vi "append to kpro data array 2016.vi"(6 "Cluster in":T1, 7 "Zeroed Pressure":dbl format="%.2f", 9 "Flow":dbl, 10 "Corrected Array in":dbl[][](array[numeric]), 11 "Feet of\nStainless to be\nUsed (Count) in":i32) -> (1 "IK":dbl, 2 "Array":dbl[][](array[numeric]), 3 "Cluster out 2":T1)   [LabVIEW 2016]
uses:
  Waterloo DAQ/controls/Kpro hydraulic measurement cluster.ctl
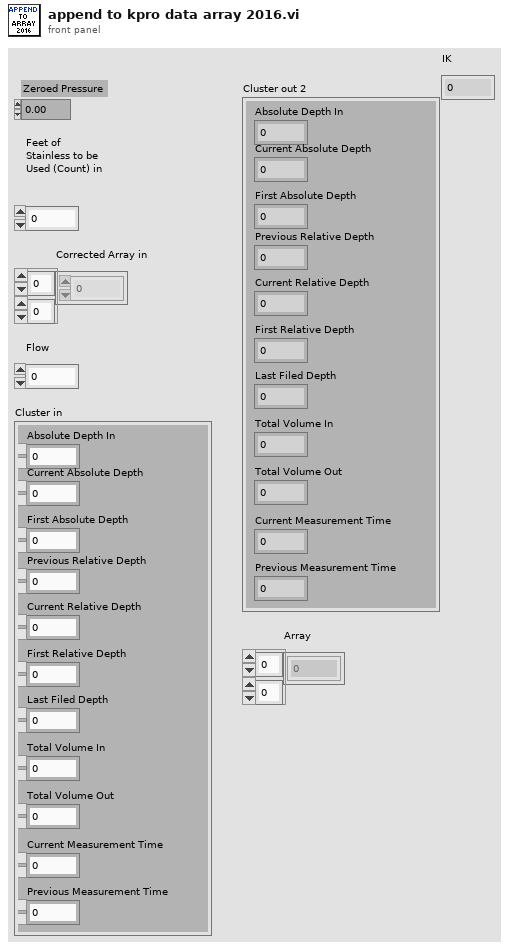
[diagram p1: front panel]
types:
  T1 = typedef "Kpro hydraulic measurement cluster.ctl" = cluster{"Absolute Depth In":dbl, "Current Absolute Depth":dbl, "First Absolute Depth":dbl, "Previous Relative Depth":dbl, "Current Relative Depth":dbl, "First Relative Depth":dbl, "Last Filed Depth":dbl, "Total Volume In":dbl, "Total Volume Out":dbl, "Current Measurement Time":dbl, "Previous Measurement Time":dbl}
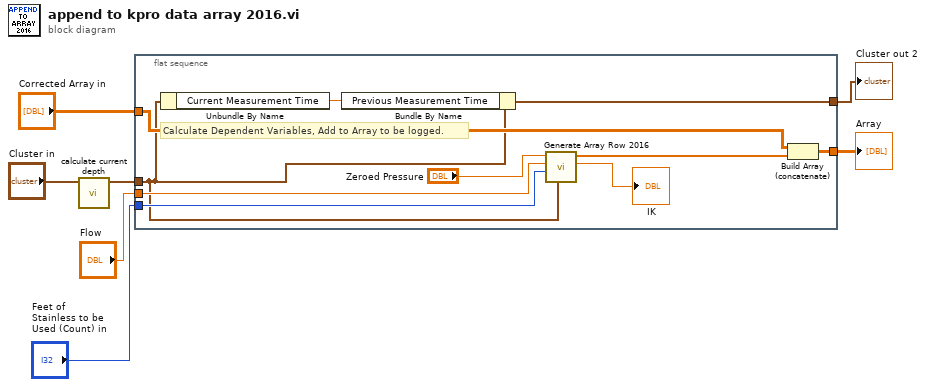
[diagram p0: block diagram]
diagram:
  n1 = call "calculate current depth.vi"("Cluster in"="Cluster in") -> ("Cluster out"=w7:T1)  [unwired: 10 in]
  n2 = flat-sequence {
    tunnel: "Corrected Array in" -> [w17]
    tunnel: [w16] -> w2
    tunnel: "Feet of\nStainless to be\nUsed (Count) in" -> [w14]
    tunnel: "Flow" -> [w13]
    tunnel: w7 -> [w11]
    tunnel: [w9] -> w5
    frame #0 {
      # "Calculate Dependent Variables, Add to Array to be logged."
      n3 = Unbundle By Name(w11) -> ("Current Measurement Time"=w10:dbl)
      n4 = Bundle By Name(cluster=w11, "Previous Measurement Time"=w10) -> (w9:T1)
      n5 = call "Generate Array Row 2016.vi"("Cluster"=w11, "Feet of\nStainless to be\nUsed (Count)"=w14, "Flow"=w13, "Zeroed Pressure"="Zeroed Pressure") -> ("IK"=→"IK":dbl, "Array"=w15:dbl[])  [unwired: 6 in]
      n6 = Build Array (concatenate)(w17, w15) -> (w16:dbl[][])
    }
  }
  "Cluster out 2" <- w5
  "Array" <- w2
